vi "GEA2_RQST_SOFTWARE_VER.vi"(0 "ComPort":refnum<visa-resource-name>="COM1", 11 "Error In":errorcluster) -> (4 "ACK":bool, 6 "Software Version":string, 10 "CRC Match":bool, 15 "Error Out":errorcluster)   [LabVIEW 2009]
uses:
  HEWH Command Type.ctl
panel:
  in  "Retries Allowed":i32=10
  out "DataReturned":u8[](array[numeric]) format="%.0x"
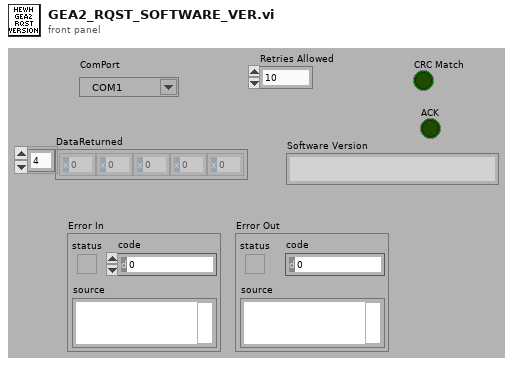
[diagram p1: front panel]
types:
  T1 = typedef "HEWH Command Type.ctl" = u8
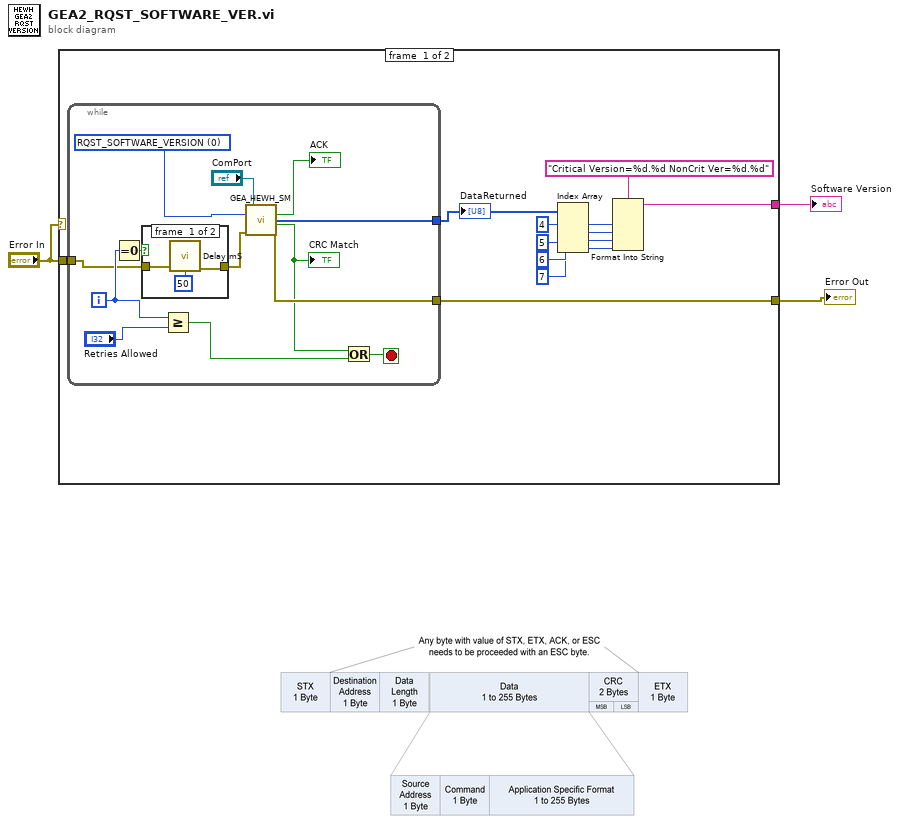
[diagram p0: block diagram]
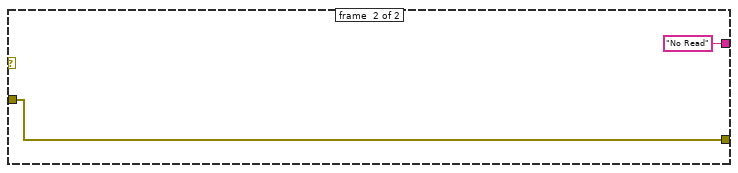
[diagram p3: hidden frame]
diagram:
  n1 = case shown="No Error" "Error In" {
    tunnel: "Error In" -> [w16 w35]
    tunnel: [w5 "No Read"] -> w3
    tunnel: [w4 w35] -> w1
    frame #0 {
      n2 = while {
        tunnel: w16 -> [w18]
        tunnel: [w27] -> w13
        tunnel: [w26] -> w4
        i -> [w20]
        stop <- w22 stop-if-true
        w17 = T1 0 items=["RQST_SOFTWARE_VERSION", "RQST_T2_RESISTANCE", "RQST_T3A_RESISTANCE", "RQST_T3B_RESISTANCE", "RQST_T4_RESISTANCE", "RQST_T5_RESISTANCE", "RQST_IDLB_RESISTANCE", "RQST_MODE_SELECT_RESISTANCE", "RQST_DATA_FROM_MEMORY", "RQST_DATA_FROM_DATA_FLASH", "RQST_SS_FAULT_COUNTS", "RQST_OTHER_FAULT_COUNTS", "CMD_CLEAR_FAULT_COUNTS", "RQST_HYPERTERM_OUTPUT_DATA", "CMD_RESET_FILTER_TIMES", "CMD_WRITE_SETPOINTS", "CMD_TURN_ON_OFF_DLB", "CMD_ENTER_EXIT_FCT_MODE", "CMD_SET_LEDS", "CMD_SET_EEV_DRIVE_LINES", "REQ_READ_KEY_STATUS", "RQST_READ_PERSONALITY", "CMD_ENTER_FACT_MODE", "CMD_RESET", "CMD_RESTORE_EEPROM_DEFAULTS", "CMD_SET_MODEL_NUMBER", "CMD_SET_SERIAL_NUMBER", "RQST_MODEL_NUMBER", "RQST_SERIAL_NUMBER", "CMD_TOGGLE_SERVICE_MODE", "CMD_TOGGLE_UE_SERV", "CMD_TOGGLE_LE_SERV", "CMD_REFRESH_SERVICE_TIMEOUTS", "RQST_DSM_OVERRIDE_STATUS", "RQST_STATUS_QUERY", "RQST_HEM_KWH_DATA", "RQST_SERVICE_ERROR_CODES", "RQST_OVERRIDE_STATUS", "CMD_UPDATE_DSM_LEVEL", "CMD_OVERRIDE_STATUS_CHANGED", "CMD_CLEAR_OVERRIDE_STATUS", "CMD_CLEAR_ENERGY_USAGE_CTRS", "CMD_DSM_OVERRIDES", "CMD_UPDATE_MODE", "CMD_SET_PID_P_DENOMINATOR", "CMD_SET_PID_I_DENOM_UNDER_THR", "CMD_SET_PID_I_DENOM_OVER_THR", "CMD_SET_START_POS_UNDER_THR", "CMD_SET_START_POS_OVER_THR", "CMD_SET_EEV_STOP_POSITION", "CMD_SET_AMBIENT_THRESH_1", "CMD_SET_AMBIENT_THRESH_2", "CMD_SET_AMBIENT_THRESH_3", "CMD_SET_PID_LOW_SH_TARGET", "CMD_SET_PID_MID_SH_TARGET", "RQST_PID_PARAMETERS", "CMD_COMP_OFF", "CMD_TOGGLE_FAN", "CMD_RQST_LED_STATUS", "CMD_UE_2_SECONDS", "CMD_LE_2_SECONDS", "CMD_COMP_ON", "CMD_HP_RUN_6MIN", "RQST_TEMP_RANGE", "RQST_VACATION_RANGE", "RQST_STD_ELEC_RANGE", "RQST_WATER_CAPACITY", "CMD_CANCEL_EEV_POSITION", "CMD_EEV_POSITION", "CMD_SET_CURRENTS", "RQST_SUPPORTED_MODES"] ("Command")
        n3 = Equal To 0?(x=w20) -> (x = 0?=w21:bool)
        n4 = case shown="False" w21 {
          tunnel: [w31 w33] -> w19
          tunnel: w18 -> [w32 w33]
          frame #0 {
            n5 = call "Delay mS.vi"("Error In"=w32, "milliseconds to wait"=u32 50) -> ("Error Out"=w31:errorcluster)  [unwired: 13 in]
          }
          frame #1 {
          }
        }
        n6 = Greater Or Equal?(x=w20, y="Retries Allowed") -> (x >= y?=w23:bool)
        n7 = call "GEA_HEWH_SM.vi"("ComPort"="ComPort", "Command"=w17, "Error In"=w19) -> ("Read_ACK"=→"ACK":bool, "DataReturned"=w27:u8[], "CRC Match"=w24:bool, "Error Out"=w26:errorcluster)  [unwired: 8 in, 1 out]
        "CRC Match" <- w24
        n8 = Or(x=w24, y=w23) -> (x .or. y?=w22:bool)
      }
      "DataReturned" <- w13
      n9 = Index Array(array=w13, index #1=4 ("index"), index #2=5 ("index"), index #3=6 ("index"), index #4=7 ("index")) -> (element #1=w15:u8, element #2=w9:u8, element #3=w8:u8, element #4=w7:u8)
      n10 = Format Into String(format string="Critical Version=%d.%d NonCrit Ver=%d.%d", w15, w9, w8, w7) -> (resulting string=w5:string)  [unwired: 2 in, 1 out]
    }
    frame #1 {
    }
  }
  "Software Version" <- w3
  "Error Out" <- w1
